vi "Coordinate_rotation.vi"(0 "Model       Roll      Pitch       Yaw (deg)":dbl[](array[numeric]) format="%#.2f", 3 "Input Position":dbl[](array[numeric]), 4 "Mode":T1(ring)) -> (5 "Output Position":dbl[](array[numeric]), 6 "Error String":string)   [LabVIEW 2011]
uses:
  <vilib>/Utility/error.llb/DialogType.ctl
  <vilib>/Analysis/coordinate.llb/Euler Rotation Order.ctl
  <vilib>/Analysis/coordinate.llb/3D Cartesian Coordinate Rotation (Euler) (Scalar).vi
  <vilib>/Analysis/NI_AALPro.lvlib
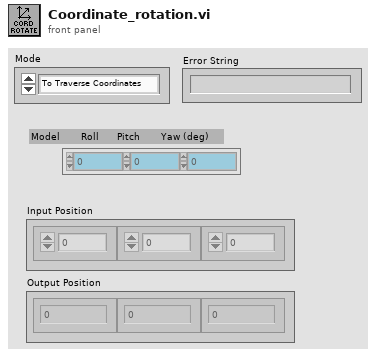
[diagram p1: front panel]
types:
  T1 = enum16{"To Traverse Coordinates", "To User Coordinates"}
  T2 = typedef "DialogType.ctl" = u16
  T3 = typedef "NI_AALPro.lvlib/Euler Rotation Order.ctl" = u16
  T4 = cluster{"Model Yaw (Deg)":dbl, "Model Yaw (Deg)":dbl, "Model Yaw (Deg)":dbl}
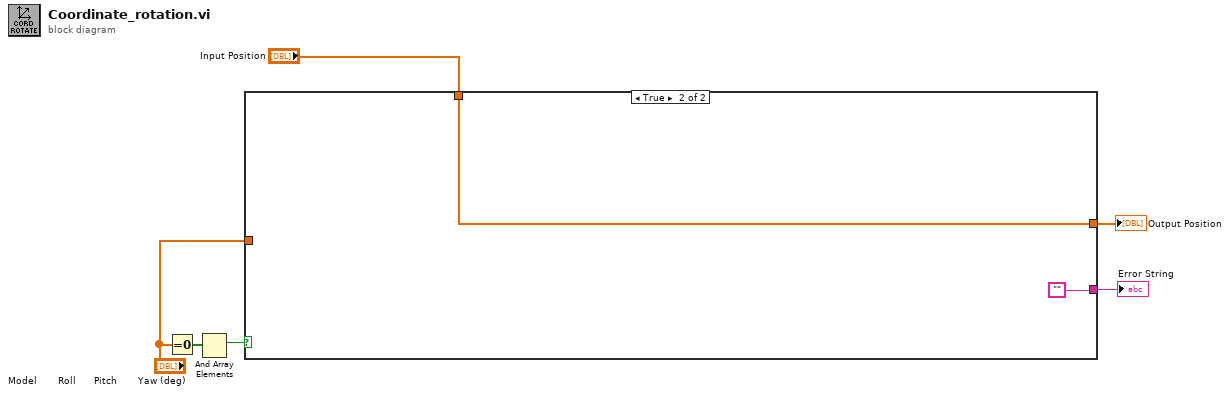
[diagram p0: block diagram]
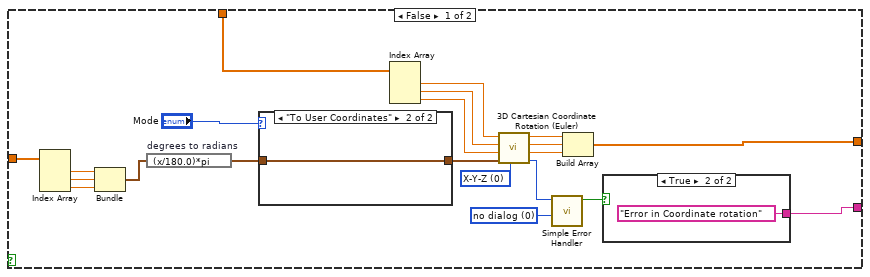
[diagram p2: hidden frame]
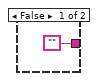
[diagram p3: hidden frame]
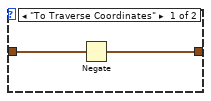
[diagram p4: hidden frame]
diagram:
  n1 = Equal To 0?(x="Model       Roll      Pitch       Yaw (deg)") -> (x = 0?=w2:bool[])
  n2 = And Array Elements(Boolean array=w2) -> (logical AND=w1:bool)
  n3 = case shown="True" w1 {
    tunnel: "Input Position" -> [w23 w34]
    tunnel: [w15 w34] -> w5
    tunnel: [w11 ""] -> w4
    tunnel: "Model       Roll      Pitch       Yaw (deg)" -> [w7 _]
    frame False {
      w13 = T2 0 items=["no dialog", "OK message", "continue or stop message", "OK message + warnings", "continue/stop + warnings"] ("type of dialog (OK msg:1)")
      w16 = T3 0 items=["X-Y-Z", "X-Z-Y", "Y-X-Z", "Y-Z-X", "Z-X-Y", "Z-Y-X", "X-Y-X", "X-Z-X", "Y-X-Y", "Y-Z-Y", "Z-X-Z", "Z-Y-Z"] ("rotation order")
      n4 = Index Array(array=w7) -> (element #1=w10:dbl, element #2=w9:dbl, element #3=w8:dbl)  [unwired: 3 in]
      n5 = Bundle("Model Yaw (Deg)"=w10, "Model Yaw (Deg)"=w9, "Model Yaw (Deg)"=w8) -> (w24:T4)  [unwired: 1 in]
      n6 = expression code="(x/180.0)*pi" "degrees to radians"(w24) -> (w26:T4)
      n7 = case shown="\"To User Coordinates\"" "Mode" {
        tunnel: w26 -> [w31 w32]
        tunnel: [w30 w32] -> w25
        frame "To Traverse Coordinates" {
          n8 = Negate(x=w31) -> (-x=w30:T4)
        }
        frame "To User Coordinates" {
        }
      }
      n9 = Index Array(array=w23) -> (element #1=w22:dbl, element #2=w21:dbl, element #3=w20:dbl)  [unwired: 3 in]
      n10 = call-poly <vilib>:"3D Cartesian Coordinate Rotation (Euler).vi"("rotation order"=w16, "Euler Angles"=w25, "z"=w20, "y"=w21, "x"=w22) -> ("error"=w14:i32, "z out"=w17:dbl, "y out"=w18:dbl, "x out"=w19:dbl)  [unwired: 3 in]
      n11 = call <vilib>:"Simple Error Handler.vi"("error code (no error:0)"=w14, "type of dialog (OK msg:1)"=w13) -> ("error?"=w12:bool)  [unwired: 3 in, 4 out]
      n12 = Build Array(w19, w18, w17) -> (w15:dbl[])
      n13 = case shown="True" w12 {
        tunnel: ["" "Error in Coordinate rotation"] -> w11
        frame False {
        }
        frame True {
        }
      }
    }
    frame True {
    }
  }
  "Output Position" <- w5
  "Error String" <- w4
